vi "Write Pre-Addressed Observer Msgs.vi"(9 "Pre-Addressed Unsubscribe Msg":refnum<class "Unsubscribe Msg.lvclass">, 10 "Pre-Addressed Subscribe Msg":refnum<class "Subscribe Msg.lvclass">, 11 "IObserver In":refnum<class "IObserver.lvclass">) -> (3 "IObserver Out":refnum<class "IObserver.lvclass">)   [LabVIEW 2015, in "IObserver.lvlib" / "IObserver.lvclass"]
doc: "<License>\nCopyright © 2017 Composed Systems, LLC | All rights reserved\nwww.composed.io\n\nAuthor: Ethan Stern <ethan.stern@composed.io>\n\nThis software is provided \"AS IS\" WITHOUT WARRANTIES, either express or implied, AND IS FOR EDUCATIONAL PURPOSES ONLY.\n</License>"
uses:
  IObserver.lvclass
  IMediator/IMediator Messages/Subscribe Msg/Subscribe Msg.lvclass
  IMediator/IMediator Messages/Unsubscribe Msg/Unsubscribe Msg.lvclass
  IObserver.lvclass/IObserver.ctl
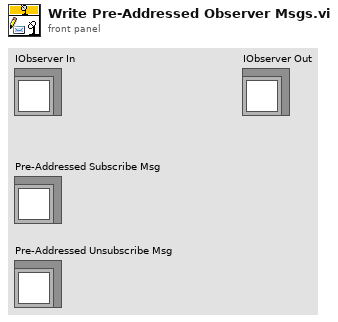
[diagram p1: front panel]
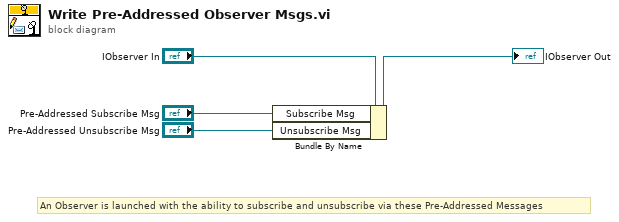
[diagram p0: block diagram]
diagram:
  # "An Observer is launched with the ability to subscribe and unsubscribe via these Pre-Addressed Messages"
  n1 = Bundle By Name(cluster="IObserver In", "Subscribe Msg"="Pre-Addressed Subscribe Msg", "Unsubscribe Msg"="Pre-Addressed Unsubscribe Msg") -> (→"IObserver Out":refnum<class "IObserver.lvclass">)
